vi "CRYUnflatten Messages.vi"(11 "Unflatten Messages":string) -> (0 "Error?":bool, 2 "Messages":T1={"Name"="Default", "Type"=0, "Command Msg"="<Enter message or command here>", "Flags"=0, "Dialog?"=FALSE, "Numeric?"=FALSE, "Wait?"=FALSE, "Pause [ms]"=0, "pattern"=0, "Address"="", "Operation"=0, "bytes"=0, "Line selected"=0, "RS232 Func"=0, "Serial Ctrl lines"=0, "Interf #"=0, "GPIB func"=0, "GPIB cmd"=0, "GPIB rem en"=FALSE, "GPIB term"=0, "Curves generated"=[], "Units"={"unit"="", "dB ref"=0.0, "axis"=0, "data"=0, "Common dB ref."=1}, "Axis"=0, "Default Value"=0.0, "Message Tilte"="", "Port #"=0, "Print Unit"="", "Text Format"={"Size"=0, "Plain"=FALSE, "Bold"=FALSE, "Italic"=FALSE, "Underline"=FALSE, "Strikethrough"=FALSE, "Color"=0, "Font"=""}, "Help"="", "Tab Value"=enum."Setting", "pattern 2"=0, "Line selected 2"=0, "H_Bits"=[], "G_Bits"=[]} {"pattern 2" format="%.0b"; "Units"."Common dB ref." items=["dB", "dBSPL", "dBPa", "dBV", "dBm", "dBu", "dBFS"]; "Units"."dB ref" format="%.2f"; "pattern" format="%.0b"; "Flags" items=["Pass", "Fail"]}, 3 "Header info":T2={"Data type"="Data            ", "Version"=1, "Dimensions"=0})   [LabVIEW 2013]
uses:
  Typedef Control/CRYMessages Cluster.ctl
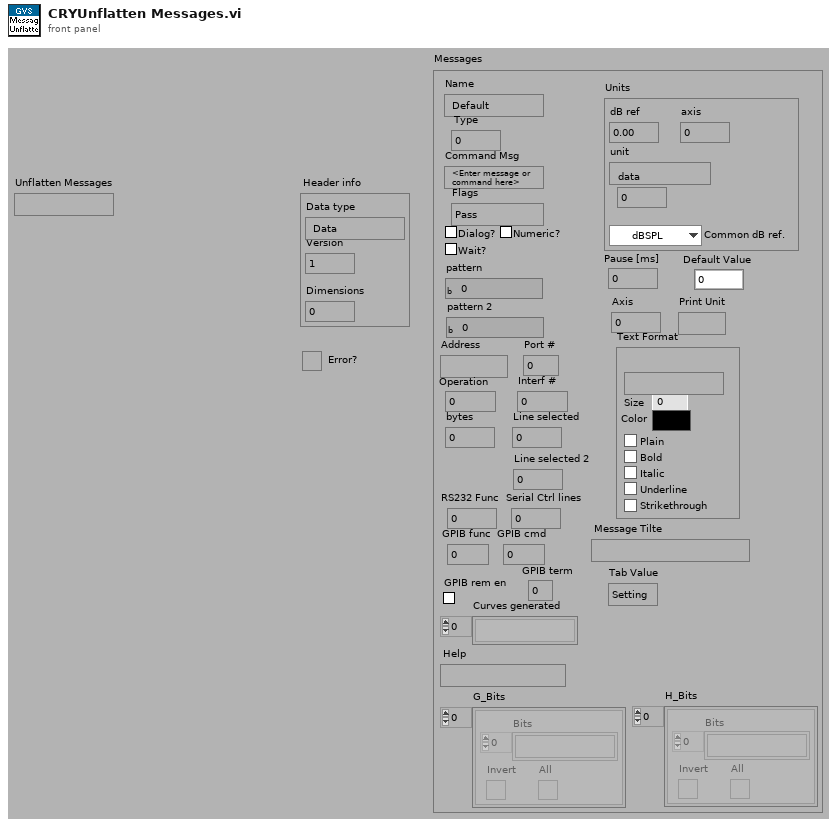
[diagram p1: front panel]
types:
  T1 = typedef "CRYMessages Cluster.ctl" = cluster{"Name":string, "Type":u16, "Command Msg":string, "Flags":u16, "Dialog?":bool, "Numeric?":bool, "Wait?":bool, "Pause [ms]":i32, "pattern":u32, "Address":string, "Operation":i32, "bytes":i32, "Line selected":u32, "RS232 Func":u16, "Serial Ctrl lines":u16, "Interf #":u8, "GPIB func":u16, "GPIB cmd":u16, "GPIB rem en":bool, "GPIB term":i32, "Curves generated":string[], "Units":cluster{"unit":string, "dB ref":dbl, "axis":u16, "data":u16, "Common dB ref.":u16}, "Axis":u16, "Default Value":dbl, "Message Tilte":string, "Port #":i32, "Print Unit":string, "Text Format":cluster{"Size":u32, "Plain":bool, "Bold":bool, "Italic":bool, "Underline":bool, "Strikethrough":bool, "Color":u32, "Font":string}, "Help":string, "Tab Value":enum32{"Setting", "Help"}, "pattern 2":u32, "Line selected 2":u32, "H_Bits":cluster{"Bits":string[], "Invert":bool, "All":bool}[], "G_Bits":cluster{"Bits":string[], "Invert":bool, "All":bool}[]}
  T2 = cluster{"Data type":string, "Version":u16, "Dimensions":u8}
  T3 = cluster{"Bits":string[], "Invert":bool, "All":bool}
  T4 = cluster{"Name":string, "Type":u16, "Command Msg":string, "Flags":u16, "Dialog?":bool, "Numeric?":bool, "Wait?":bool, "Pause [ms]":i32, "pattern":u32, "Address":string, "Operation":i32, "bytes":i32, "Line selected":u32, "RS232 Func":u16, "Serial Ctrl lines":u16, "Interf #":u8, "GPIB func":u16, "GPIB cmd":u16, "GPIB rem en":bool, "GPIB term":i32, "Curves generated":string[], "Units":cluster{"unit":string, "dB ref":dbl, "axis":u16, "data":u16, "Common dB ref.":u16}, "Axis":u16, "Default Value":dbl, "Message Tilte":string, "Port #":i32, "Print Unit":string, "Text Format":cluster{"Size":u32, "Plain":bool, "Bold":bool, "Italic":bool, "Underline":bool, "Strikethrough":bool, "Color":u32, "Font":string}, "Help":string, "Tab Value":enum32{"Setting", "Help"}, "pattern 2":u32, "Line selected 2":u32, "H_Bits":cluster{"Bits":string[], "Invert":bool, "All":bool}[], "G_Bits":cluster{"Bits":string[], "Invert":bool, "All":bool}[]}
  T5 = cluster{"unsigned byte array[0]":u8, "unsigned byte array[1]":u8, "unsigned byte array[2]":u8}
  T6 = cluster{"Name":string, "Type":u16, "Command Msg":string, "Flags":u16, "Dialog?":bool, "Numeric?":bool, "Wait?":bool, "Pause [ms]":i32, "pattern":u32, "Address":string, "Operation":i32, "bytes":i32, "Line selected":u32, "RS232 Func":u16, "Serial Ctrl lines":u16, "Interf #":u8, "GPIB func":u16, "GPIB cmd":u16, "GPIB rem en":bool, "GPIB term":i32, "Curves generated":string[], "Units":cluster{"unit":string, "dB ref":dbl, "axis":u16, "data":u16, "Common dB ref.":u16}, "Axis":u16, "Default Value":dbl, "Message Tilte":string, "Port #":i32, "Print Unit":string, "Text Format":cluster{"Size":u32, "Plain":bool, "Bold":bool, "Italic":bool, "Underline":bool, "Strikethrough":bool, "Font":u16, "Color":u32}}
  T7 = cluster{"unit":string, "dB ref":dbl, "axis":u16, "data":u16, "Common dB ref.":u16}
  T8 = cluster{"Name":string, "Type":u16, "Command Msg":string, "Flags":u16, "Dialog?":bool, "Numeric?":bool, "Wait?":bool, "Pause [ms]":i32, "pattern":u32, "Address":string, "Operation":i32, "bytes":i32, "Line selected":u32, "RS232 Func":u16, "Serial Ctrl lines":u16, "Interf #":u8, "GPIB func":u16, "GPIB cmd":u16, "GPIB rem en":bool, "GPIB term":i32, "Curves generated":string[], "Units":cluster{"unit":string, "dB ref":dbl, "axis":u16, "data":u16, "Common dB ref.":u16}, "Axis":u16, "Default Value":dbl, "Message Tilte":string, "Port #":i32, "Print Unit":string, "Text Format":cluster{"Size":u32, "Plain":bool, "Bold":bool, "Italic":bool, "Underline":bool, "Strikethrough":bool, "Color":u32, "Font":string}}
  T9 = cluster{"Name":string, "Type":u16, "Command Msg":string, "Flags":u16, "Dialog?":bool, "Numeric?":bool, "Wait?":bool, "Pause [ms]":i32, "pattern":u32, "Address":string, "Operation":i32, "bytes":i32, "Line selected":u32, "RS232 Func":u16, "Serial Ctrl lines":u16, "Interf #":u8, "GPIB func":u16, "GPIB cmd":u16, "GPIB rem en":bool, "GPIB term":i32, "Curves generated":string[], "Units":cluster{"unit":string, "dB ref":dbl, "axis":u16, "data":u16, "Common dB ref.":u16}, "Axis":u16, "Default Value":dbl, "Message Tilte":string, "Port #":i32, "Print Unit":string, "Text Format":cluster{"Size":u32, "Plain":bool, "Bold":bool, "Italic":bool, "Underline":bool, "Strikethrough":bool, "Color":u32, "Font":string}, "Help":string, "Tab Value":enum32{"Setting", "Help"}}
  T10 = cluster{"Name":string, "Type":u16, "Command Msg":string, "Flags":u16, "Dialog?":bool, "Numeric?":bool, "Wait?":bool, "Pause [ms]":i32, "pattern":u32, "Address":string, "Operation":i32, "bytes":i32, "Line selected":u32, "RS232 Func":u16, "Serial Ctrl lines":u16, "Interf #":u8, "GPIB func":u16, "GPIB cmd":u16, "GPIB rem en":bool, "GPIB term":i32, "Curves generated":string[], "Units":cluster{"unit":string, "dB ref":dbl, "axis":u16, "data":u16, "Common dB ref.":u16}, "Axis":u16, "Default Value":dbl, "Message Tilte":string, "Port #":i32, "Print Unit":string, "Text Format":cluster{"Size":u32, "Plain":bool, "Bold":bool, "Italic":bool, "Underline":bool, "Strikethrough":bool, "Color":u32, "Font":string}, "Help":string, "Tab Value":enum32{"Setting", "Help"}, "pattern 2":u32, "Line selected 2":u32}
  T11 = cluster{"substring":string, u16, "unsigned byte array[2]":u8}
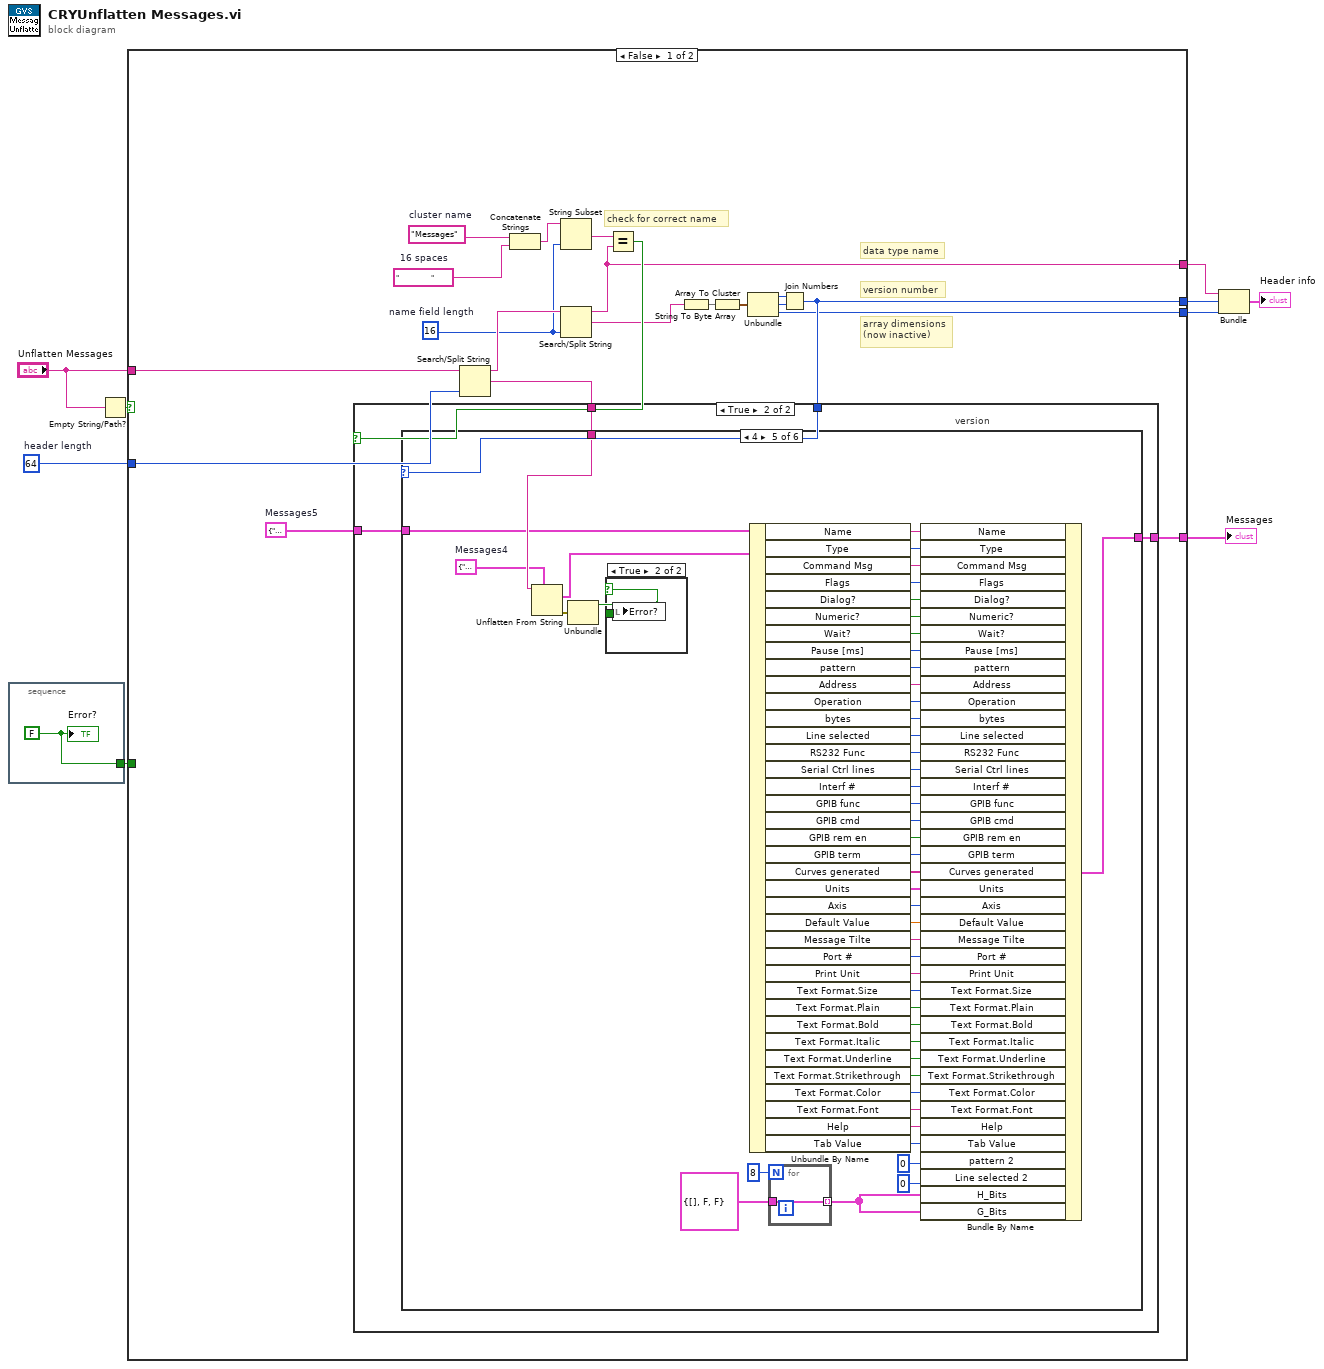
[diagram p0: block diagram]
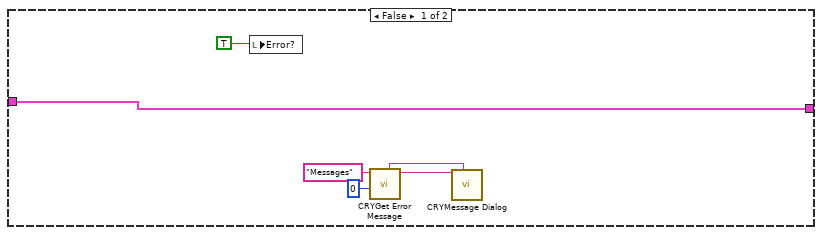
[diagram p2: hidden frame]
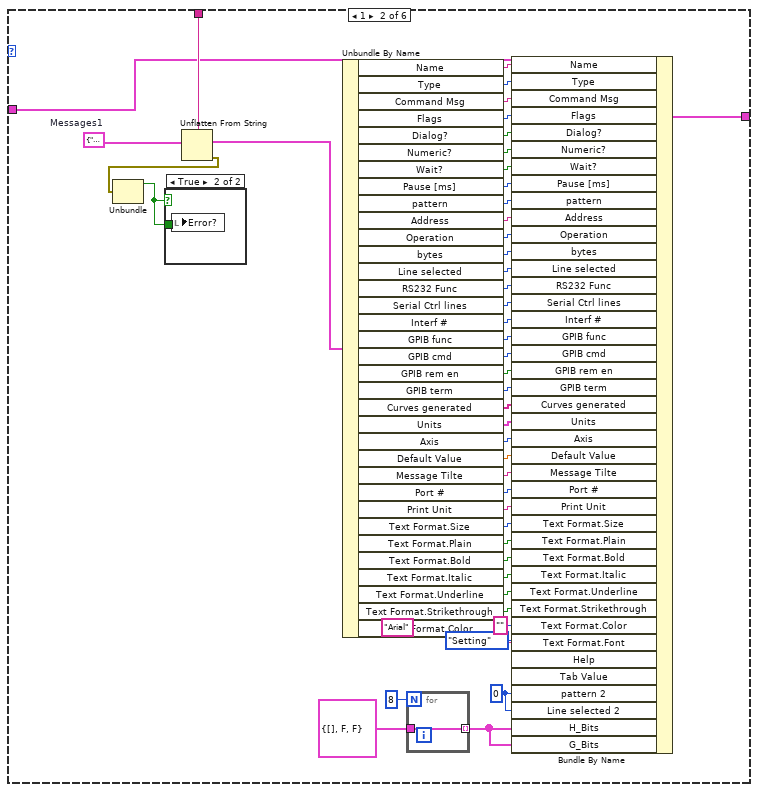
[diagram p4: hidden frame]
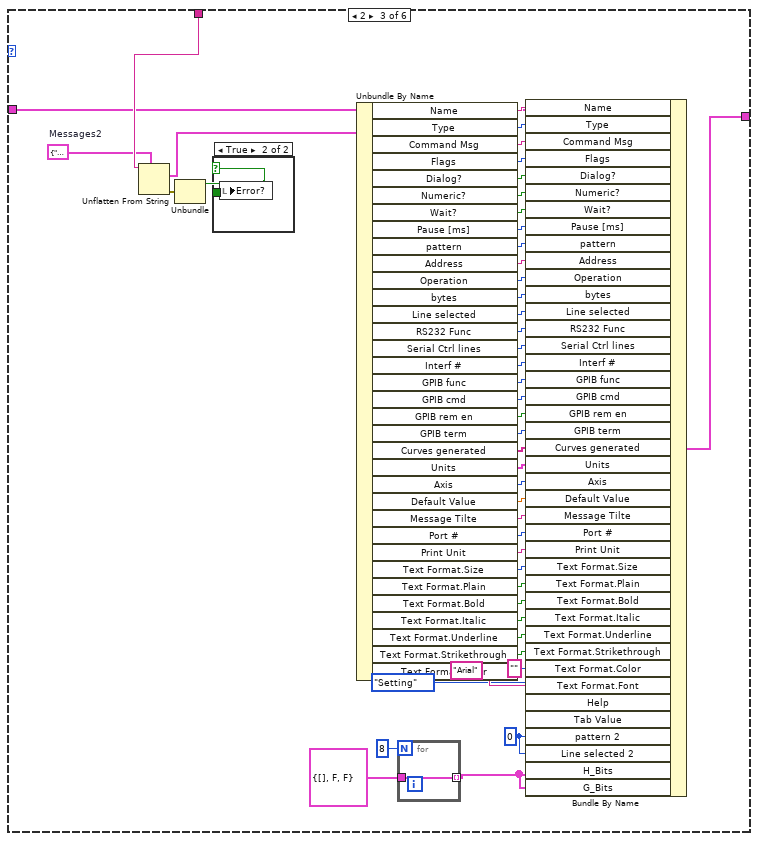
[diagram p6: hidden frame]
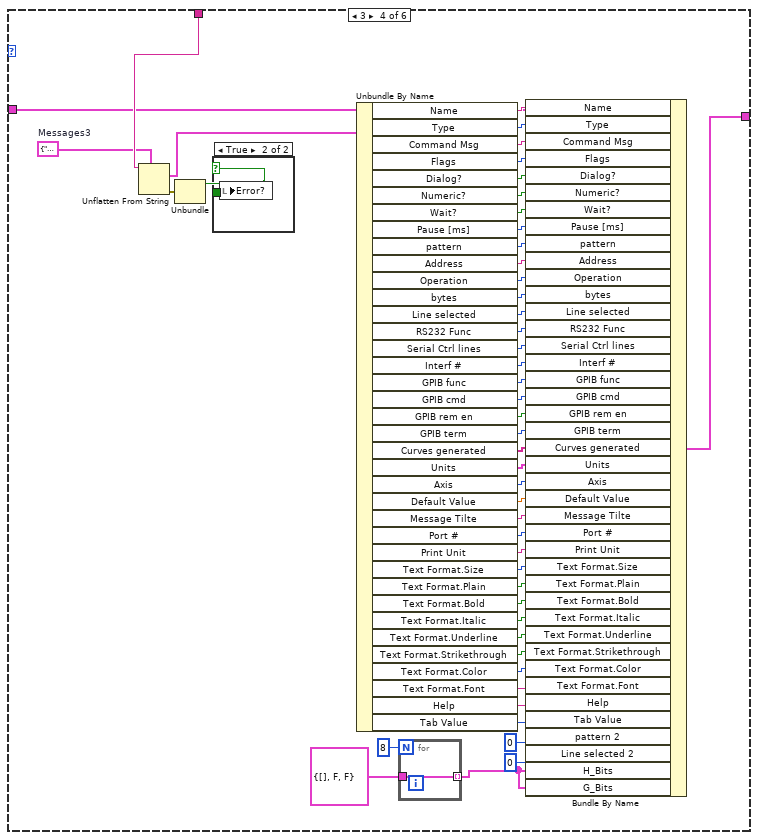
[diagram p8: hidden frame]
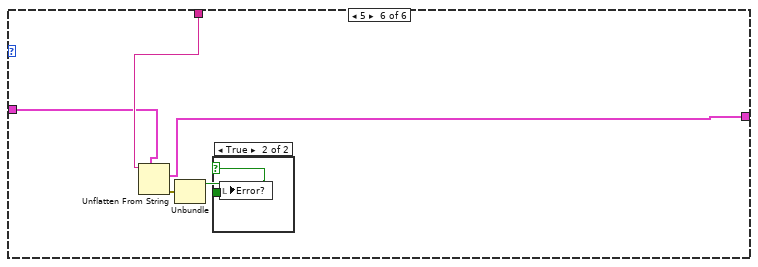
[diagram p11: hidden frame]
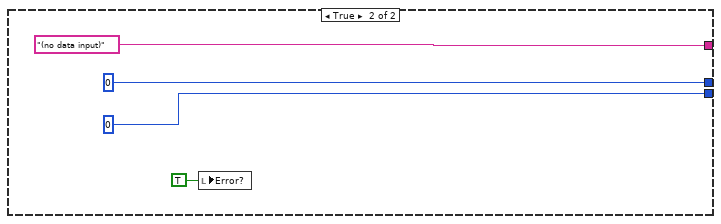
[diagram p13: hidden frame]
diagram:
  w7 = 64  # header length
  n1 = stacked-sequence {
    tunnel: [w10] -> w2
    frame #0 {
      w10 = FALSE
      "Error?" <- w10
    }
  }
  n2 = Empty String/Path?(string/path="Unflatten Messages") -> (empty?=w8:bool)
  n3 = case shown="False" w8 {
    tunnel: "Unflatten Messages" -> [w30 _]
    tunnel: w7 -> [w24 _]
    tunnel: [w21 u16 0] -> w5
    tunnel: [w13 u8 0] -> w6
    tunnel: [w14 "(no data input)" ("substring")] -> w4
    tunnel: w2 -> [_ _]
    tunnel: [w12 _] -> w1
    frame False {
      w11 = T4 {"Name"="Default", "Type"=0, "Command Msg"="<Enter message or command here>", "Flags"=0, "Dialog?"=FALSE, "Numeric?"=FALSE, "Wait?"=FALSE, "Pause [ms]"=0, "pattern"=0, "Address"="", "Operation"=0, "bytes"=0, "Line selected"=0, "RS232 Func"=0, "Serial Ctrl lines"=0, "Interf #"=0, "GPIB func"=0, "GPIB cmd"=0, "GPIB rem en"=FALSE, "GPIB term"=0, "Curves generated"=[], "Units"={"unit"="", "dB ref"=0.0, "axis"=0, "data"=0, "Common dB ref."=1}, "Axis"=0, "Default Value"=0.0, "Message Tilte"="", "Port #"=0, "Print Unit"="", "Text Format"={"Size"=0, "Plain"=FALSE, "Bold"=FALSE, "Italic"=FALSE, "Underline"=FALSE, "Strikethrough"=FALSE, "Color"=0, "Font"=""}, "Help"="", "Tab Value"=enum."Setting", "pattern 2"=0, "Line selected 2"=0, "H_Bits"=[], "G_Bits"=[]}  # Messages5
      w18 = "                "  # 16 spaces
      w19 = "Messages"  # cluster name
      w16 = 16  # name field length
      # "check for correct name"
      # "array dimensions\n(now inactive)"
      # "version number"
      # "data type name"
      n4 = Search/Split String(string=w30, offset (0)=w24) -> (substring before match=w23:string, match + rest of string=w25:string)  [unwired: 2 out]
      n5 = Concatenate Strings(w19, w18) -> (w17:string)
      n6 = String Subset(string=w17, length (rest)=w16) -> (substring=w15:string)  [unwired: 1 out]
      n7 = Search/Split String(string=w23, offset (0)=w16) -> (substring before match=w14:string, match + rest of string=w20:string)  [unwired: 2 out]
      n8 = Equal?(x=w15, y=w14) -> (x = y?=w22:bool)
      n9 = String To Byte Array(string=w20) -> (unsigned byte array=w29:u8[])
      n10 = Array To Cluster(array=w29) -> (cluster=w28:T5)
      n11 = Unbundle(w28) -> ("unsigned byte array[0]"=w27:u8, "unsigned byte array[1]"=w26:u8, "unsigned byte array[2]"=w13:u8)
      n12 = Join Numbers(hi=w27, lo=w26) -> ((hi.lo)=w21:u16)
      n13 = case shown="True" w22 {
        tunnel: w25 -> [_ w40]
        tunnel: w21 -> [_ w39]
        tunnel: [w35 w38] -> w12
        tunnel: w11 -> [w35 w37]
        frame False {
          n14 = local write "Error?"(TRUE) -> ()
          n15 = call "CRYGet Error Message.vi"("Error No"=0 ("No"), "Kind"="Messages") -> ("Message"=w31:string, "Window Title"=w32:string)  [unwired: 4 in, 4 out]
          n16 = call "CRYMessage Dialog.vi"("Window Title"=w32, "Message Content"=w31) -> ()  [unwired: 8 in, 2 out]
        }
        frame True {
          n17 = case "version" shown="4" w39 {
            tunnel: w40 -> [_ w89 w137 w188 w239 w246]
            tunnel: [w41 w56 w97 w151 w202 w244] -> w38
            tunnel: w37 -> [w41 w84 w98 w152 w203 w245]
            frame Default {
            }
            frame 1 {
              w45 = u32 0 ("pattern 2")
              w86 = T6 {"Name"="", "Type"=0, "Command Msg"="", "Flags"=0, "Dialog?"=FALSE, "Numeric?"=FALSE, "Wait?"=FALSE, "Pause [ms]"=0, "pattern"=0, "Address"="", "Operation"=0, "bytes"=0, "Line selected"=0, "RS232 Func"=0, "Serial Ctrl lines"=0, "Interf #"=0, "GPIB func"=0, "GPIB cmd"=0, "GPIB rem en"=FALSE, "GPIB term"=0, "Curves generated"=[], "Units"={"unit"="", "dB ref"=0.0, "axis"=0, "data"=0, "Common dB ref."=0}, "Axis"=0, "Default Value"=0.0, "Message Tilte"="", "Port #"=0, "Print Unit"="", "Text Format"={"Size"=0, "Plain"=FALSE, "Bold"=FALSE, "Italic"=FALSE, "Underline"=FALSE, "Strikethrough"=FALSE, "Font"=0, "Color"=0}}  # Messages1
              n18 = Unflatten From String(type=w86, binary string=w89) -> (value=w85:T6, error out=w87:errorcluster)  [unwired: 1 in, 3 out]
              n19 = Unbundle(w87) -> ("status"=w88:bool)  [unwired: 2 out]
              n20 = case shown="True" w88 {
                tunnel: w88 -> [_ w91]
                frame False {
                }
                frame True {
                  n21 = local write "Error?"(w91) -> ()
                }
              }
              n22 = Unbundle By Name(w85) -> ("Name"=w83:string, "Type"=w82:u16, "Command Msg"=w81:string, "Flags"=w80:u16, "Dialog?"=w79:bool, "Numeric?"=w78:bool, "Wait?"=w77:bool, "Pause [ms]"=w76:i32, "pattern"=w75:u32, "Address"=w74:string, "Operation"=w73:i32, "bytes"=w72:i32, "Line selected"=w71:u32, "RS232 Func"=w70:u16, "Serial Ctrl lines"=w69:u16, "Interf #"=w68:u8, "GPIB func"=w67:u16, "GPIB cmd"=w66:u16, "GPIB rem en"=w65:bool, "GPIB term"=w64:i32, "Curves generated"=w63:string[], "Units"=w62:T7, "Axis"=w61:u16, "Default Value"=w60:dbl, "Message Tilte"=w59:string, "Port #"=w58:i32, "Print Unit"=w57:string, "Text Format.Size"=w55:u32, "Text Format.Plain"=w54:bool, "Text Format.Bold"=w53:bool, "Text Format.Italic"=w52:bool, "Text Format.Underline"=w51:bool, "Text Format.Strikethrough"=w50:bool, "Text Format.Color"=w49:u32)
              n23 = for {
                N: 8 -> [_]
                tunnel: T3 {"Bits"=[], "Invert"=FALSE, "All"=FALSE} ("Element") -> [w90]
                tunnel: [w90] -> w42 mode=indexing
              }
              n24 = Bundle By Name(cluster=w84, "Name"=w83, "Type"=w82, "Command Msg"=w81, "Flags"=w80, "Dialog?"=w79, "Numeric?"=w78, "Wait?"=w77, "Pause [ms]"=w76, "pattern"=w75, "Address"=w74, "Operation"=w73, "bytes"=w72, "Line selected"=w71, "RS232 Func"=w70, "Serial Ctrl lines"=w69, "Interf #"=w68, "GPIB func"=w67, "GPIB cmd"=w66, "GPIB rem en"=w65, "GPIB term"=w64, "Curves generated"=w63, "Units"=w62, "Axis"=w61, "Default Value"=w60, "Message Tilte"=w59, "Port #"=w58, "Print Unit"=w57, "Text Format.Size"=w55, "Text Format.Plain"=w54, "Text Format.Bold"=w53, "Text Format.Italic"=w52, "Text Format.Underline"=w51, "Text Format.Strikethrough"=w50, "Text Format.Color"=w49, "Text Format.Font"="Arial", "Help"="", "Tab Value"=enum32{"Setting", "Help"}."Setting", "pattern 2"=w45, "Line selected 2"=w45, "H_Bits"=w42, "G_Bits"=w42) -> (w56:T4)
            }
            frame 2 {
              w95 = u32 0 ("pattern 2")
              w136 = T8 {"Name"="Default", "Type"=0, "Command Msg"="<Enter message or command here>", "Flags"=0, "Dialog?"=FALSE, "Numeric?"=FALSE, "Wait?"=FALSE, "Pause [ms]"=0, "pattern"=0, "Address"="", "Operation"=0, "bytes"=0, "Line selected"=0, "RS232 Func"=0, "Serial Ctrl lines"=0, "Interf #"=0, "GPIB func"=0, "GPIB cmd"=0, "GPIB rem en"=FALSE, "GPIB term"=0, "Curves generated"=[], "Units"={"unit"="", "dB ref"=0.0, "axis"=0, "data"=0, "Common dB ref."=1}, "Axis"=0, "Default Value"=0.0, "Message Tilte"="", "Port #"=0, "Print Unit"="", "Text Format"={"Size"=0, "Plain"=FALSE, "Bold"=FALSE, "Italic"=FALSE, "Underline"=FALSE, "Strikethrough"=FALSE, "Color"=0, "Font"=""}}  # Messages2
              n25 = Unflatten From String(type=w136, binary string=w137) -> (value=w99:T8, error out=w138:errorcluster)  [unwired: 1 in, 3 out]
              n26 = Unbundle(w138) -> ("status"=w139:bool)  [unwired: 2 out]
              n27 = case shown="True" w139 {
                tunnel: w139 -> [_ w141]
                frame False {
                }
                frame True {
                  n28 = local write "Error?"(w141) -> ()
                }
              }
              n29 = Unbundle By Name(w99) -> ("Name"=w135:string, "Type"=w134:u16, "Command Msg"=w133:string, "Flags"=w132:u16, "Dialog?"=w131:bool, "Numeric?"=w130:bool, "Wait?"=w129:bool, "Pause [ms]"=w128:i32, "pattern"=w127:u32, "Address"=w126:string, "Operation"=w125:i32, "bytes"=w124:i32, "Line selected"=w123:u32, "RS232 Func"=w122:u16, "Serial Ctrl lines"=w121:u16, "Interf #"=w120:u8, "GPIB func"=w119:u16, "GPIB cmd"=w118:u16, "GPIB rem en"=w117:bool, "GPIB term"=w116:i32, "Curves generated"=w115:string[], "Units"=w114:T7, "Axis"=w113:u16, "Default Value"=w112:dbl, "Message Tilte"=w111:string, "Port #"=w110:i32, "Print Unit"=w109:string, "Text Format.Size"=w108:u32, "Text Format.Plain"=w107:bool, "Text Format.Bold"=w106:bool, "Text Format.Italic"=w105:bool, "Text Format.Underline"=w104:bool, "Text Format.Strikethrough"=w103:bool, "Text Format.Color"=w102:u32)
              n30 = for {
                N: 8 -> [_]
                tunnel: T3 {"Bits"=[], "Invert"=FALSE, "All"=FALSE} ("Element") -> [w140]
                tunnel: [w140] -> w92 mode=indexing
              }
              n31 = Bundle By Name(cluster=w98, "Name"=w135, "Type"=w134, "Command Msg"=w133, "Flags"=w132, "Dialog?"=w131, "Numeric?"=w130, "Wait?"=w129, "Pause [ms]"=w128, "pattern"=w127, "Address"=w126, "Operation"=w125, "bytes"=w124, "Line selected"=w123, "RS232 Func"=w122, "Serial Ctrl lines"=w121, "Interf #"=w120, "GPIB func"=w119, "GPIB cmd"=w118, "GPIB rem en"=w117, "GPIB term"=w116, "Curves generated"=w115, "Units"=w114, "Axis"=w113, "Default Value"=w112, "Message Tilte"=w111, "Port #"=w110, "Print Unit"=w109, "Text Format.Size"=w108, "Text Format.Plain"=w107, "Text Format.Bold"=w106, "Text Format.Italic"=w105, "Text Format.Underline"=w104, "Text Format.Strikethrough"=w103, "Text Format.Color"=w102, "Text Format.Font"="Arial", "Help"="", "Tab Value"=enum32{"Setting", "Help"}."Setting", "pattern 2"=w95, "Line selected 2"=w95, "H_Bits"=w92, "G_Bits"=w92) -> (w97:T4)
            }
            frame 3 {
              w150 = T9 {"Name"="Default", "Type"=0, "Command Msg"="<Enter message or command here>", "Flags"=0, "Dialog?"=FALSE, "Numeric?"=FALSE, "Wait?"=FALSE, "Pause [ms]"=0, "pattern"=0, "Address"="", "Operation"=0, "bytes"=0, "Line selected"=0, "RS232 Func"=0, "Serial Ctrl lines"=0, "Interf #"=0, "GPIB func"=0, "GPIB cmd"=0, "GPIB rem en"=FALSE, "GPIB term"=0, "Curves generated"=[], "Units"={"unit"="", "dB ref"=0.0, "axis"=0, "data"=0, "Common dB ref."=1}, "Axis"=0, "Default Value"=0.0, "Message Tilte"="", "Port #"=0, "Print Unit"="", "Text Format"={"Size"=0, "Plain"=FALSE, "Bold"=FALSE, "Italic"=FALSE, "Underline"=FALSE, "Strikethrough"=FALSE, "Color"=0, "Font"=""}, "Help"="", "Tab Value"=enum."Setting"}  # Messages3
              n32 = Unflatten From String(type=w150, binary string=w188) -> (value=w153:T9, error out=w189:errorcluster)  [unwired: 1 in, 3 out]
              n33 = Unbundle(w189) -> ("status"=w190:bool)  [unwired: 2 out]
              n34 = case shown="True" w190 {
                tunnel: w190 -> [_ w192]
                frame False {
                }
                frame True {
                  n35 = local write "Error?"(w192) -> ()
                }
              }
              n36 = Unbundle By Name(w153) -> ("Name"=w187:string, "Type"=w186:u16, "Command Msg"=w185:string, "Flags"=w184:u16, "Dialog?"=w183:bool, "Numeric?"=w182:bool, "Wait?"=w181:bool, "Pause [ms]"=w180:i32, "pattern"=w179:u32, "Address"=w178:string, "Operation"=w177:i32, "bytes"=w176:i32, "Line selected"=w175:u32, "RS232 Func"=w174:u16, "Serial Ctrl lines"=w173:u16, "Interf #"=w172:u8, "GPIB func"=w171:u16, "GPIB cmd"=w170:u16, "GPIB rem en"=w169:bool, "GPIB term"=w168:i32, "Curves generated"=w167:string[], "Units"=w166:T7, "Axis"=w165:u16, "Default Value"=w164:dbl, "Message Tilte"=w163:string, "Port #"=w162:i32, "Print Unit"=w161:string, "Text Format.Size"=w160:u32, "Text Format.Plain"=w159:bool, "Text Format.Bold"=w158:bool, "Text Format.Italic"=w157:bool, "Text Format.Underline"=w156:bool, "Text Format.Strikethrough"=w155:bool, "Text Format.Color"=w154:u32, "Text Format.Font"=w149:string, "Help"=w148:string, "Tab Value"=w147:enum32{"Setting", "Help"})
              n37 = for {
                N: 8 -> [_]
                tunnel: T3 {"Bits"=[], "Invert"=FALSE, "All"=FALSE} ("Element") -> [w191]
                tunnel: [w191] -> w142 mode=indexing
              }
              n38 = Bundle By Name(cluster=w152, "Name"=w187, "Type"=w186, "Command Msg"=w185, "Flags"=w184, "Dialog?"=w183, "Numeric?"=w182, "Wait?"=w181, "Pause [ms]"=w180, "pattern"=w179, "Address"=w178, "Operation"=w177, "bytes"=w176, "Line selected"=w175, "RS232 Func"=w174, "Serial Ctrl lines"=w173, "Interf #"=w172, "GPIB func"=w171, "GPIB cmd"=w170, "GPIB rem en"=w169, "GPIB term"=w168, "Curves generated"=w167, "Units"=w166, "Axis"=w165, "Default Value"=w164, "Message Tilte"=w163, "Port #"=w162, "Print Unit"=w161, "Text Format.Size"=w160, "Text Format.Plain"=w159, "Text Format.Bold"=w158, "Text Format.Italic"=w157, "Text Format.Underline"=w156, "Text Format.Strikethrough"=w155, "Text Format.Color"=w154, "Text Format.Font"=w149, "Help"=w148, "Tab Value"=w147, "pattern 2"=u32 0, "Line selected 2"=u32 0, "H_Bits"=w142, "G_Bits"=w142) -> (w151:T4)
            }
            frame 4 {
              w196 = T10 {"Name"="Default", "Type"=0, "Command Msg"="<Enter message or command here>", "Flags"=0, "Dialog?"=FALSE, "Numeric?"=FALSE, "Wait?"=FALSE, "Pause [ms]"=0, "pattern"=0, "Address"="", "Operation"=0, "bytes"=0, "Line selected"=0, "RS232 Func"=0, "Serial Ctrl lines"=0, "Interf #"=0, "GPIB func"=0, "GPIB cmd"=0, "GPIB rem en"=FALSE, "GPIB term"=0, "Curves generated"=[], "Units"={"unit"="", "dB ref"=0.0, "axis"=0, "data"=0, "Common dB ref."=1}, "Axis"=0, "Default Value"=0.0, "Message Tilte"="", "Port #"=0, "Print Unit"="", "Text Format"={"Size"=0, "Plain"=FALSE, "Bold"=FALSE, "Italic"=FALSE, "Underline"=FALSE, "Strikethrough"=FALSE, "Color"=0, "Font"=""}, "Help"="", "Tab Value"=enum."Setting", "pattern 2"=0, "Line selected 2"=0}  # Messages4
              n39 = Unflatten From String(type=w196, binary string=w239) -> (value=w204:T10, error out=w240:errorcluster)  [unwired: 1 in, 3 out]
              n40 = Unbundle(w240) -> ("status"=w241:bool)  [unwired: 2 out]
              n41 = case shown="True" w241 {
                tunnel: w241 -> [_ w243]
                frame False {
                }
                frame True {
                  n42 = local write "Error?"(w243) -> ()
                }
              }
              n43 = Unbundle By Name(w204) -> ("Name"=w238:string, "Type"=w237:u16, "Command Msg"=w236:string, "Flags"=w235:u16, "Dialog?"=w234:bool, "Numeric?"=w233:bool, "Wait?"=w232:bool, "Pause [ms]"=w231:i32, "pattern"=w230:u32, "Address"=w229:string, "Operation"=w228:i32, "bytes"=w227:i32, "Line selected"=w226:u32, "RS232 Func"=w225:u16, "Serial Ctrl lines"=w224:u16, "Interf #"=w223:u8, "GPIB func"=w222:u16, "GPIB cmd"=w221:u16, "GPIB rem en"=w220:bool, "GPIB term"=w219:i32, "Curves generated"=w218:string[], "Units"=w217:T7, "Axis"=w216:u16, "Default Value"=w215:dbl, "Message Tilte"=w214:string, "Port #"=w213:i32, "Print Unit"=w212:string, "Text Format.Size"=w211:u32, "Text Format.Plain"=w210:bool, "Text Format.Bold"=w209:bool, "Text Format.Italic"=w208:bool, "Text Format.Underline"=w207:bool, "Text Format.Strikethrough"=w206:bool, "Text Format.Color"=w205:u32, "Text Format.Font"=w201:string, "Help"=w200:string, "Tab Value"=w199:enum32{"Setting", "Help"})
              n44 = for {
                N: 8 -> [_]
                tunnel: T3 {"Bits"=[], "Invert"=FALSE, "All"=FALSE} ("Element") -> [w242]
                tunnel: [w242] -> w193 mode=indexing
              }
              n45 = Bundle By Name(cluster=w203, "Name"=w238, "Type"=w237, "Command Msg"=w236, "Flags"=w235, "Dialog?"=w234, "Numeric?"=w233, "Wait?"=w232, "Pause [ms]"=w231, "pattern"=w230, "Address"=w229, "Operation"=w228, "bytes"=w227, "Line selected"=w226, "RS232 Func"=w225, "Serial Ctrl lines"=w224, "Interf #"=w223, "GPIB func"=w222, "GPIB cmd"=w221, "GPIB rem en"=w220, "GPIB term"=w219, "Curves generated"=w218, "Units"=w217, "Axis"=w216, "Default Value"=w215, "Message Tilte"=w214, "Port #"=w213, "Print Unit"=w212, "Text Format.Size"=w211, "Text Format.Plain"=w210, "Text Format.Bold"=w209, "Text Format.Italic"=w208, "Text Format.Underline"=w207, "Text Format.Strikethrough"=w206, "Text Format.Color"=w205, "Text Format.Font"=w201, "Help"=w200, "Tab Value"=w199, "pattern 2"=u32 0, "Line selected 2"=u32 0, "H_Bits"=w193, "G_Bits"=w193) -> (w202:T4)
            }
            frame 5 {
              n46 = Unflatten From String(type=w245, binary string=w246) -> (value=w244:T4, error out=w247:errorcluster)  [unwired: 1 in, 3 out]
              n47 = Unbundle(w247) -> ("status"=w248:bool)  [unwired: 2 out]
              n48 = case shown="True" w248 {
                tunnel: w248 -> [_ w249]
                frame False {
                }
                frame True {
                  n49 = local write "Error?"(w249) -> ()
                }
              }
            }
          }
        }
      }
    }
    frame True {
      n50 = local write "Error?"(TRUE ("Error?")) -> ()
    }
  }
  "Messages" <- w1
  n51 = Bundle("substring"=w4, w5, "unsigned byte array[2]"=w6) -> (→"Header info":T11)  [unwired: 1 out]
